vi "brushbar_info.vi"(6 "timeout (25000ms)":i32=25000, 8 "error in (no error)":errorcluster, 11 "daemon reference in":refnum<k5>) -> (0 "error out":errorcluster, 1 "brushbar data":T1, 2 "response":string, 3 "daemon reference out":refnum<k5>, 5 "command out":string="random")   [LabVIEW 2017]
doc: "<b>Command: </b>\"template\"\n\n<b>Description: </b> This command does something.\n\n<b>Parameters: </b> None\n____________________________________________\nDIPC 692 Daemon API 10.0.0.1\nSam Tee - Dyson Technology Ltd\nCopyright (c) 2024, Dyson Technology Ltd"
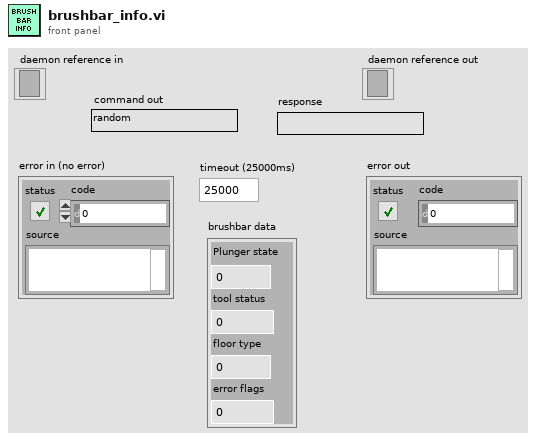
[diagram p1: front panel]
types:
  T1 = cluster{"Plunger state":dbl, "tool status":dbl, "floor type":dbl, "error flags":dbl}
  T2 = cluster{"array type (2D Dbl)[0]":dbl, "array type (2D Dbl)[1]":dbl, "array type (2D Dbl)[2]":dbl, "array type (2D Dbl)[3]":dbl}
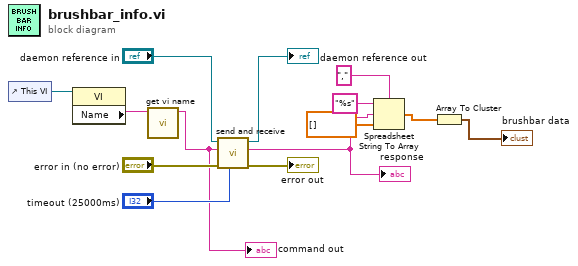
[diagram p0: block diagram]
diagram:
  n1 = control-ref of="This VI"() -> (w9:refnum<vi>)
  n2 = property class="VI"(reference=w9) -> ("Name"=w8:string)  [unwired: 1 in, 2 out]
  n3 = call "get vi name.vi"("library.lvlib:name.vi"=w8) -> ("vi name"=w7:string)  [unwired: 10 in]
  "command out" <- w7
  n4 = call "send and receive.vi"("timeout (25000ms)"="timeout (25000ms)", "error in (no error)"="error in (no error)", "command"=w7, "daemon reference in"="daemon reference in") -> ("error out"=→"error out":errorcluster, "response"=w4:string, "daemon reference out"=→"daemon reference out":refnum<k5>)  [unwired: 5 in]
  "response" <- w4
  n5 = Spreadsheet String To Array(delimiter (Tab)=",", format string="%s", spreadsheet string=w4, array type (2D Dbl)=dbl[] []) -> (array=w2:dbl[])
  n6 = Array To Cluster(array=w2) -> (cluster=→"brushbar data":T2)
